vi "Point Cloud Raw Test Data.vi"() -> (3 "Input UDP packet array 2":i32[][](array[numeric]))   [LabVIEW 2018]
uses:
  LiDAR.lvclass
  Controls/cls_Point_Cloud_Data.ctl
  Controls/cls_Point_Cloud_Packet_Header.ctl
  Controls/cls_Point_Cloud_Ray_Header.ctl
  Controls/cls_Point_Cloud_Return_Data.ctl
panel:
  out "Pount Cloud Data out":T1 {"Ray Header Data"."Return Data Array"."Reflectance" format="%.6f %"; "Ray Header Data"."Return Data Array"."Range" format="%.4f M"; "Ray Header Data"."Return Data Array"."Existence Probability" format="%.4f %"; "Ray Header Data"."Elevation" format="%.6f"; "Ray Header Data"."Azimuth" format="%.6f"}
  in  "LiDAR in":refnum<class "LiDAR.lvclass">
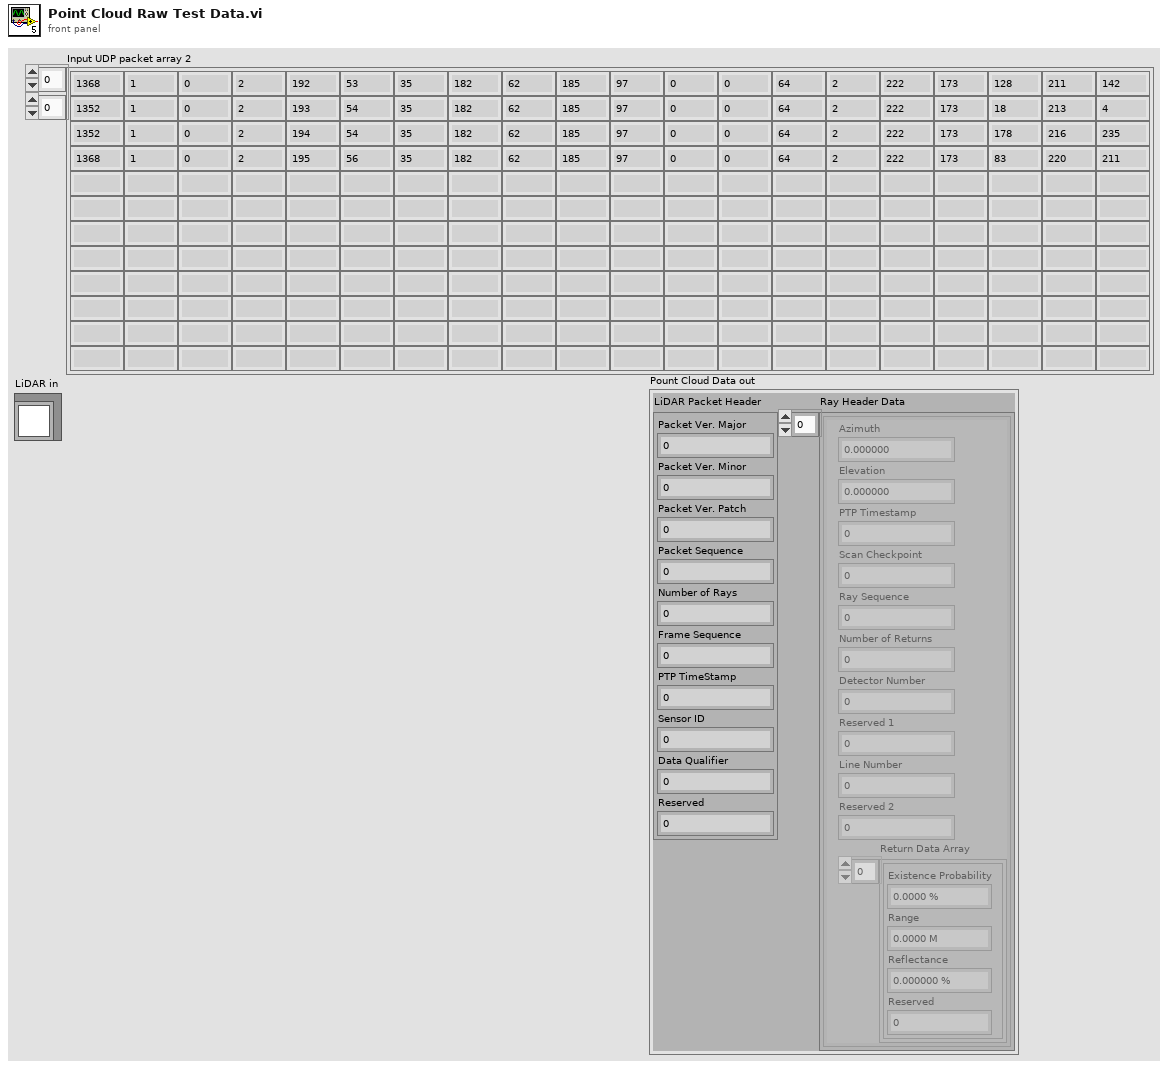
[diagram p1: front panel]
types:
  T1 = typedef "LiDAR.lvlib/LiDAR.lvclass/cls_Point_Cloud_Data.ctl" = cluster{"LiDAR Packet Header":T2, "Ray Header Data":T3[]}
  T2 = typedef "LiDAR.lvlib/LiDAR.lvclass/cls_Point_Cloud_Packet_Header.ctl" = cluster{"Packet Ver. Major":u8, "Packet Ver. Minor":u8, "Packet Ver. Patch":u8, "Packet Sequence":u8, "Number of Rays":u8, "Frame Sequence":u8, "PTP TimeStamp":u64, "Sensor ID":u8, "Data Qualifier":u8, "Reserved":u16}
  T3 = typedef "LiDAR.lvlib/LiDAR.lvclass/cls_Point_Cloud_Ray_Header.ctl" = cluster{"Azimuth":dbl, "Elevation":dbl, "PTP Timestamp":u32, "Scan Checkpoint":u8, "Ray Sequence":u8, "Number of Returns":u8, "Detector Number":u8, "Reserved 1":u8, "Line Number":u16, "Reserved 2":u32, "Return Data Array":T4[]}
  T4 = typedef "LiDAR.lvlib/LiDAR.lvclass/cls_Point_Cloud_Return_Data.ctl" = cluster{"Existence Probability":dbl, "Range":dbl, "Reflectance":dbl, "Reserved":u16}
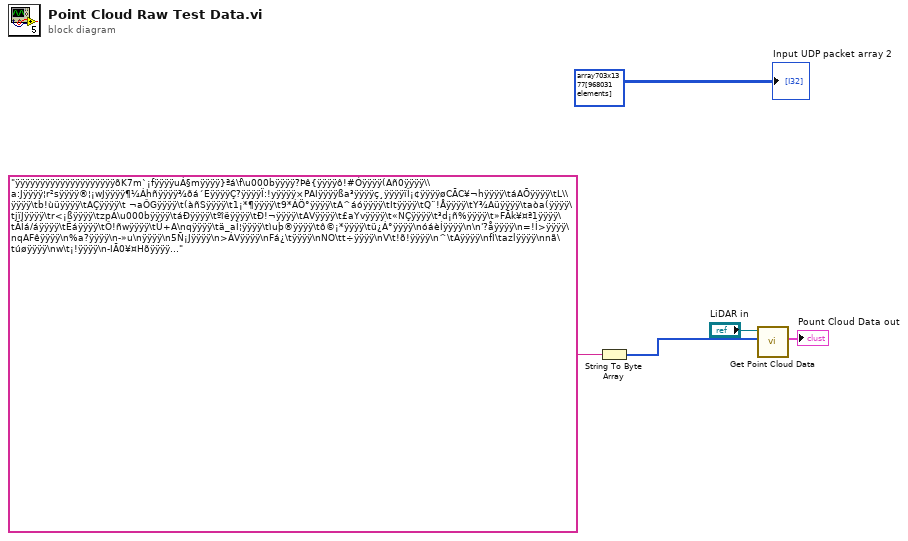
[diagram p0: block diagram]
diagram:
  n1 = String To Byte Array(string="ÿÿÿÿÿÿÿÿÿÿÿÿÿÿÿÿÿÿÿÿõK7m`¡fÿÿÿÿuÁ§mÿÿÿÿ}ªá\f\u000bÿÿÿÿ?Þê{ÿÿÿÿô!#Óÿÿÿÿ(Añ0ÿÿÿÿ\\a:Jÿÿÿÿ¦r²sÿÿÿÿ®¦¡wJÿÿÿÿ¶¼Áhñÿÿÿÿ¾ðá´EÿÿÿÿÇ?ÿÿÿÿÏ:!yÿÿÿÿ×PAIÿÿÿÿßa³ÿÿÿÿç¸ÿÿÿÿïÎ¡¢ÿÿÿÿøCÃC¥¬hÿÿÿÿ\táAÕÿÿÿÿ\tL\\ÿÿÿÿ\tb!ùüÿÿÿÿ\tAÇÿÿÿÿ\t ¬aÔGÿÿÿÿ\t(àñSÿÿÿÿ\t1¡*¶ÿÿÿÿ\t9*ÁÖ°ÿÿÿÿ\tA^áóÿÿÿÿ\tItÿÿÿÿ\tQ¨!Åÿÿÿÿ\tY¾Aüÿÿÿÿ\taòa(ÿÿÿÿ\tjïJÿÿÿÿ\tr<¡ßÿÿÿÿ\tzpÁ\u000bÿÿÿÿ\táÐÿÿÿÿ\tºîëÿÿÿÿ\tÐ!¬ÿÿÿÿ\tAVÿÿÿÿ\t£aYvÿÿÿÿ\t«NÇÿÿÿÿ\t³d¡ñ%ÿÿÿÿ\t»FÃk¥¤ª1ÿÿÿÿ\tÃÌá/áÿÿÿÿ\tËáÿÿÿÿ\tÔ!ñwÿÿÿÿ\tÜ+A\nqÿÿÿÿ\tä_aÎ¦ÿÿÿÿ\tìuþ®ÿÿÿÿ\tô©¡*ÿÿÿÿ\tü¿Á°ÿÿÿÿ\nóáèÍÿÿÿÿ\n\n'?åÿÿÿÿ\n=!Í>ÿÿÿÿ\nqAFêÿÿÿÿ\n%a?ÿÿÿÿ\n-»u\nÿÿÿÿ\n5Ñ¡Jÿÿÿÿ\n>ÁVÿÿÿÿ\nFá¿\tÿÿÿÿ\nNO\tt÷ÿÿÿÿ\nV\t!õ!ÿÿÿÿ\n^\tAÿÿÿÿ\nfÍ\tazlÿÿÿÿ\nnã\túøÿÿÿÿ\nw\t¡!ÿÿÿÿ\n-IÃ0¥¤Hõÿÿÿÿ...") -> (unsigned byte array=w3:u8[])
  n2 = call "Get Point Cloud Data.vi"("Test Data"=w3, "LiDAR in"="LiDAR in") -> ("Pount Cloud Data out"=→"Pount Cloud Data out":T1)  [unwired: 7 in, 2 out]
  "Input UDP packet array 2" <- i32[][] array703x1377[968031 elements] ("Input UDP packet array")
